vi "Read Exception Status.vi"(8 "error in (no error)":errorcluster, 11 "Modbus master in":refnum<class "Modbus Master.lvclass">) -> (0 "error out":errorcluster, 2 "exception status":u8, 3 "Modbus master out":refnum<class "Modbus Master.lvclass">)   [LabVIEW 2021, in "Modbus Master.lvclass"]
doc: "Reads the exception status of a Modbus slave. The exception status is a set of eight status bits. Each status bit represents an exception."
uses:
  Modbus Master.lvclass
  Modbus Master.lvclass/Modbus Master.ctl
  Network Protocol/Network Master/Network Master.lvclass
  Master Function Definition/Master Function Definition.lvclass
  Transmission Data Unit/Serial Interface/Serial Data Unit.lvclass
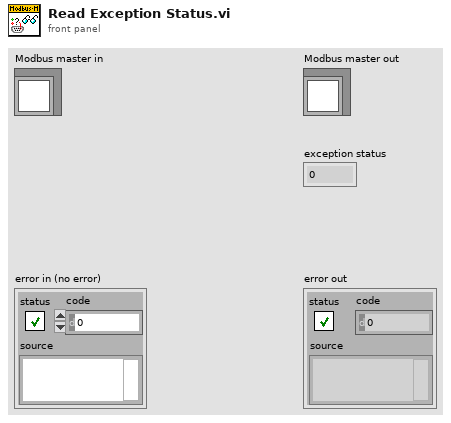
[diagram p1: front panel]
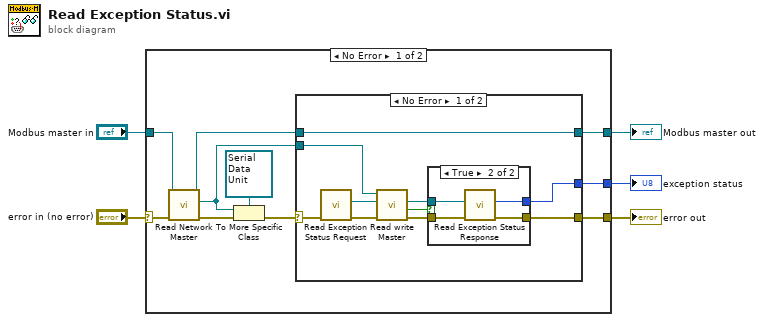
[diagram p0: block diagram]
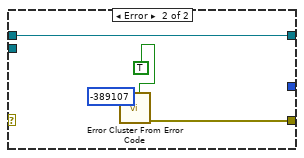
[diagram p3: hidden frame]
diagram:
  n1 = case shown="No Error" "error in (no error)" {
    selector: "error in (no error)" -> [w10 w35]
    tunnel: [w14 w36] -> w5
    tunnel: "Modbus master in" -> [w13 w36]
    tunnel: [w12 _] -> w3
    tunnel: [w11 w35] -> w2
    frame No Error {
      n2 = call "Read Network Master.vi"("error in"=w10, "Modbus master in"=w13) -> ("error out"=w9:errorcluster, "Network Master"=w8:refnum<class "Network Master.lvclass">, "Modbus master out"=w15:refnum<class "Modbus Master.lvclass">)  [unwired: 7 in]
      n3 = To More Specific Class(target class=refnum<class "Serial Data Unit.lvclass"> refnum ("Serial Data Unit"), reference=w8, error in=w9) -> (error out=w6:errorcluster)  [unwired: 1 out]
      n4 = case shown="No Error" w6 {
        selector: w6 -> [w21 _]
        tunnel: w15 -> [w20 w33]
        tunnel: [w20 w33] -> w14
        tunnel: [w24 _] -> w12
        tunnel: [w22 w34] -> w11
        tunnel: w8 -> [w18 _]
        frame No Error {
          n5 = call "Read Exception Status Request.vi"("error in"=w21) -> ("error out"=w25:errorcluster, "modbus data unit out"=w19:refnum<class "Modbus Data Unit.lvclass">)  [unwired: 9 in]
          n6 = call "Read write Master.vi"("error in (no error)"=w25, "Modbus data unit in"=w19, "Modbus master in"=w18) -> ("error out"=w23:errorcluster, "PDU valid?"=w17:bool, "Modbus data unit out"=w16:refnum<class "Modbus Data Unit.lvclass">)  [unwired: 5 in, 1 out]
          n7 = case shown="True" w17 {
            tunnel: [_ w30] -> w24
            tunnel: w16 -> [_ w29]
            tunnel: w23 -> [w26 w28]
            tunnel: [w26 w27] -> w22
            frame False {
            }
            frame True {
              n8 = call "Read Exception Status Response.vi"("error in"=w28, "modbus data unit in"=w29) -> ("error out"=w27:errorcluster, "Exception Status"=w30:u8)  [unwired: 8 in]
            }
          }
        }
        frame Error {
          n9 = call <vilib>:"Error Cluster From Error Code.vi"("is warning? (False)"=TRUE, "error code (0)"=-389107) -> ("error out"=w34:errorcluster)  [unwired: 7 in]
        }
      }
    }
    frame Error {
    }
  }
  "error out" <- w2
  "Modbus master out" <- w5
  "exception status" <- w3
